vi "Host.vi"() -> ()   [LabVIEW 2013]
uses:
  <vilib>/userdefined/High Color/nirio_resource_hc.ctl
  <instrlib>/niDCPower/nidcpower.llb/niDCPower Measurement Type.ctl
  <vilib>/FPGAPlugInAG/PXI-7953R/niLvFpga_Open_PXI-7953R.vi
  <vilib>/rvi/interface/common/dynamic/niFpgaDynamicAddResources.vi
  <vilib>/FPGAPlugInAG/Dynamic/niLvFpga_Reset_Dynamic.vi
  <vilib>/FPGAPlugInAG/Dynamic/niLvFpga_Run_Dynamic.vi
  <vilib>/rvi/interface/common/niFpgaWaitOnOcc.vi
  <vilib>/Utility/error.llb/Error Cluster From Error Code.vi
  <vilib>/rvi/errors/niLvFpgaAdjustHostInterfaceError.vi
  <vilib>/FPGAPlugInAG/Dynamic/niLvFpga_Close_Dynamic.vi
  <vilib>/rvi/interface/nirviOpenFPGA/nirviOpenFPGA.xnode
  FPGA Bitfiles/MUX1_FPGATarget_Target_25MmX6rN+ac.lvbitx
  <vilib>/rvi/interface/nirviMethod/nirviMethod.xnode
  <vilib>/rvi/interface/nirviReadWriteControl/nirviReadWriteControl.xnode
  <vilib>/rvi/interface/nirviCloseFPGA/nirviCloseFPGA.xnode
  NiFpgaLv.dll
  <vilib>/rvi/interface/Simulation/niFpgaSimulationCallBeginRW.vi
panel:
  in  "100мс до бита":u32=100
  out "СБОЙ":bool
  out "Тиристор":bool
  out "СБОИ":i32
  out "S2":bool
  out "S1":bool
  out "S0":bool
  in  "Контроль S":bool
  in  "VR_ON":bool=TRUE
  out "TST":bool
  out "VDD":i32
  out "VDD3":i32
  out "VDDO":i32
  out "VR":i32
  out "VDDA":i32
  in  "VDD3_selcur":dbl=0.04 caption="current limit" format="%_6p"
  in  "RN":bool
  in  "Автомат":bool
  out "VR":bool
  in  "SEL_Time, мс":u32=100
  in  "SIM_SEL":bool
  in  "VDDA_selcur":dbl=0.04 caption="current limit" format="%_6p"
  in  "VR_selcur":dbl=0.04 caption="current limit" format="%_6p"
  in  "VDDO_selcur":dbl=0.04 caption="current limit" format="%_6p"
  in  "VDD_selcur":dbl=0.04 caption="current limit" format="%_6p"
  in  "VDDA":dbl=3.3 caption="voltage level" format="%_6p"
  in  "VDD3":dbl=3.3 caption="voltage level" format="%_6p"
  in  "VDDA_curlim":dbl=0.05 caption="current limit" format="%_6p"
  in  "VR_curlim":dbl=0.05 caption="current limit" format="%_6p"
  in  "VDD3_curlim":dbl=0.05 caption="current limit" format="%_6p"
  in  "VDD_curlim":dbl=0.05 caption="current limit" format="%_6p"
  out "VDDA_cur":dbl caption="measurement" format="%_6g"
  out "VR_cur":dbl caption="measurement" format="%_6g"
  out "VDD3_cur":dbl caption="measurement" format="%_6g"
  out "VDD_cur":dbl caption="measurement" format="%_6g"
  in  "VR":dbl=3.0 caption="voltage level" format="%_6p"
  in  "VDD":dbl=1.3999999999999997 caption="voltage level" format="%_6p"
  in  "VDDO":dbl=3.3 caption="voltage level" format="%_6p"
  in  "VDDO_curlim":dbl=0.05 caption="current limit" format="%_6p"
  out "VDDO_cur":dbl caption="measurement" format="%_6g"
  out "VDDA":bool
  out "VDDO":bool
  out "VDD3":bool
  out "VDD":bool
  in  "Питание":bool
  in  "Стоп":bool
  in  "VDDA_VR":refnum<k15>="PXI2Slot2" caption="instrument handle"
  in  "VDDO_VDD3":refnum<k15>="PXI1Slot3" caption="instrument handle"
  in  "VDD":refnum<k15>="PXI1Slot4" caption="instrument handle"
  in  "resource name":T1="PXI1Slot5"
  in  "SEL_SEU":path=path "C:/VPL/LabView_PRJ/MUX_1 Folder/VPL/LabView_PRJ/Мультиплексор_2/LOGS"
  out "Номер образца":string="0"
  out "Температура":string="0"
  out "S2":i16
  out "S1":i16
  out "S0":i16
  # "ПЛИС"
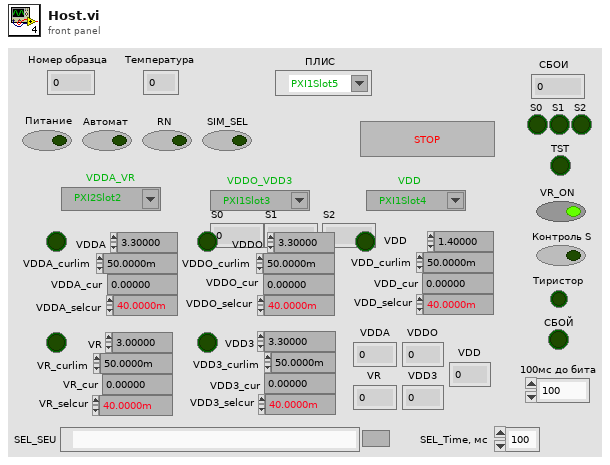
[diagram p1: front panel]
types:
  T1 = typedef "nirio_resource_hc.ctl" = tag
  T2 = enum16{"open", "replace", "create", "open or create", "replace or create", "replace or create with confirmation"}
  T3 = typedef "niDCPower Measurement Type.ctl" = i32
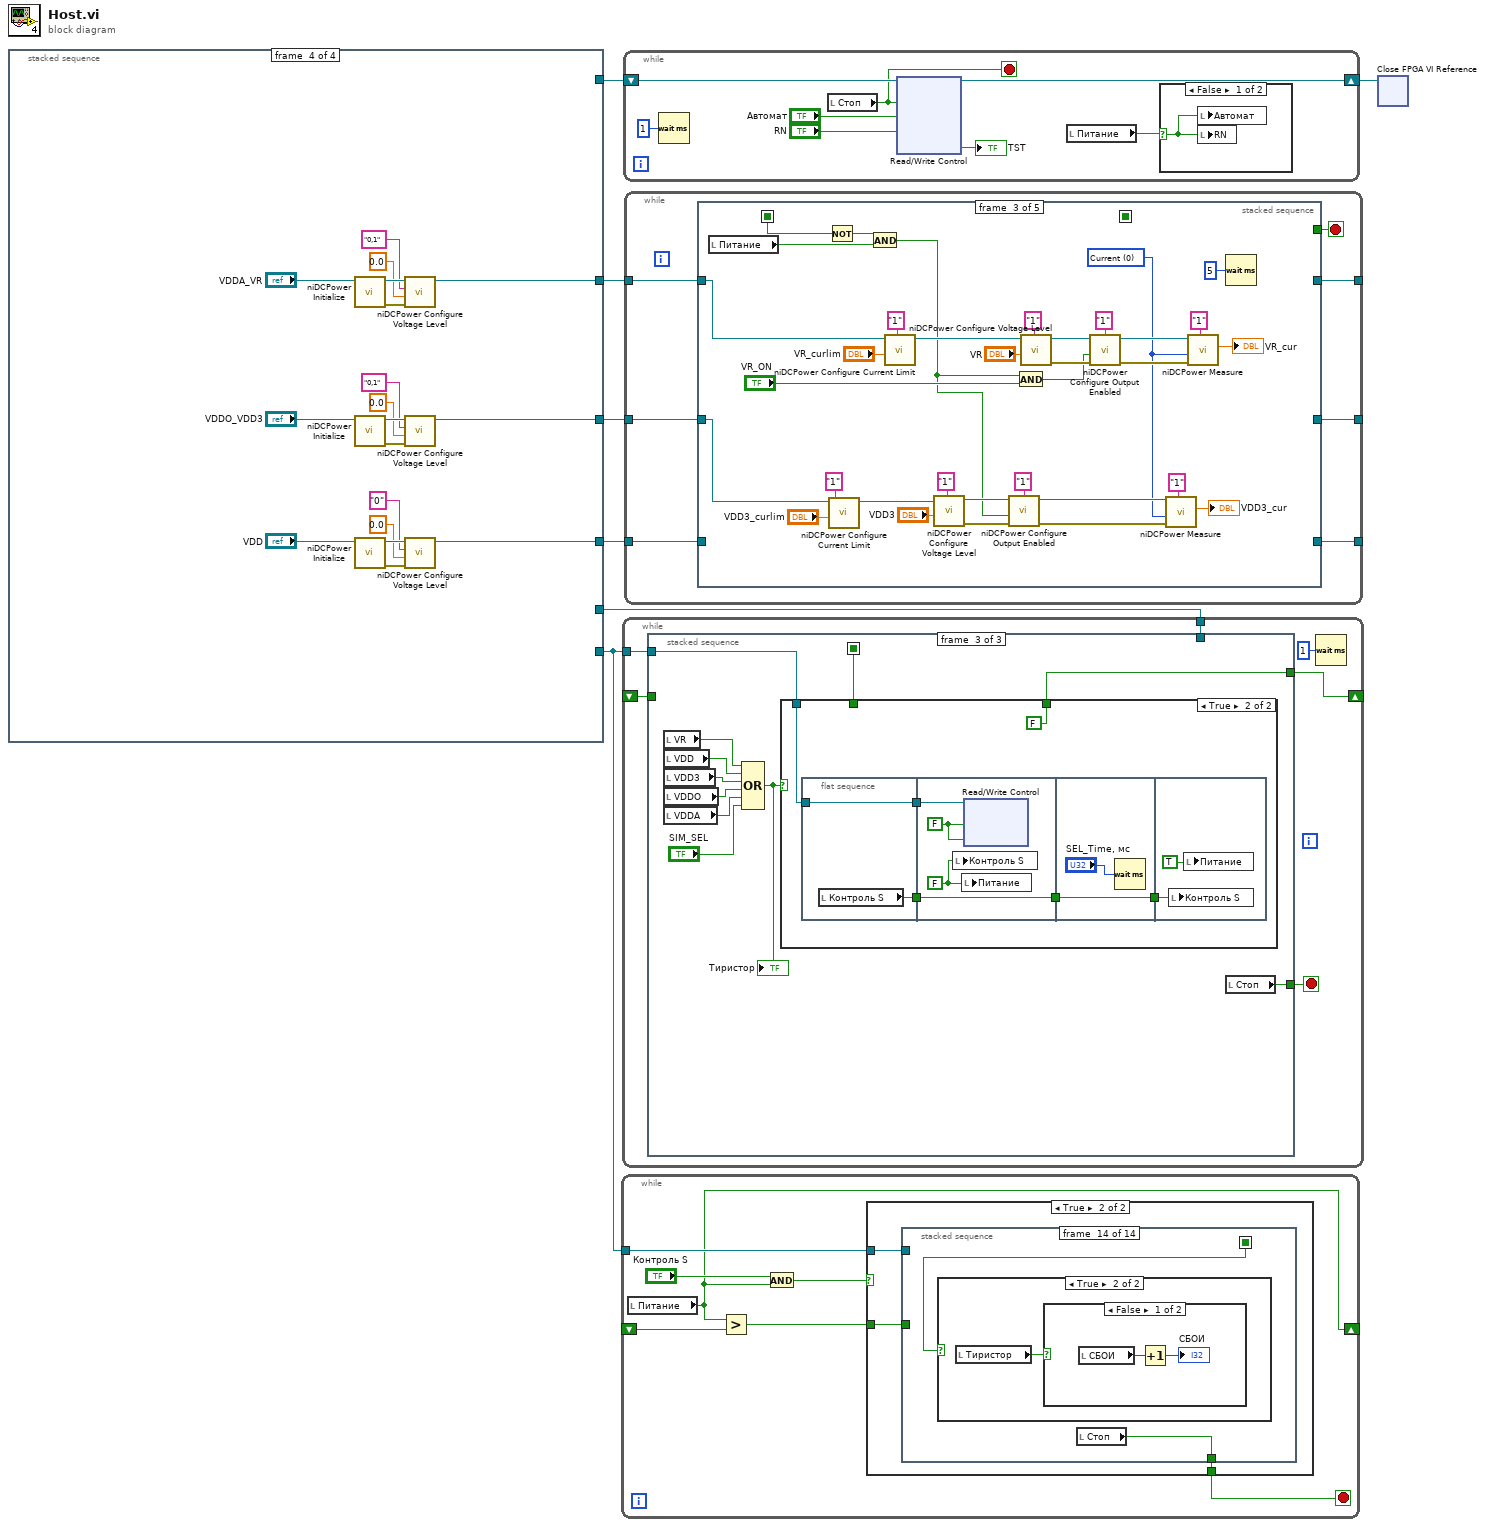
[diagram p0: block diagram]
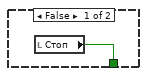
[diagram p2: hidden frame]
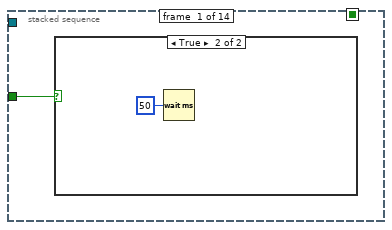
[diagram p3: hidden frame]
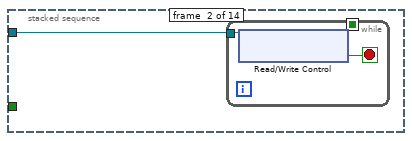
[diagram p5: hidden frame]
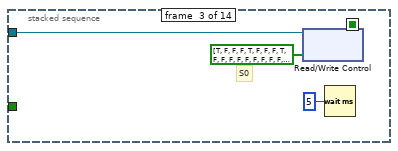
[diagram p6: hidden frame]
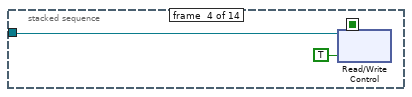
[diagram p7: hidden frame]
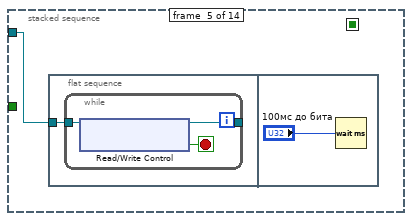
[diagram p8: hidden frame]
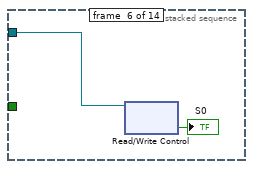
[diagram p9: hidden frame]
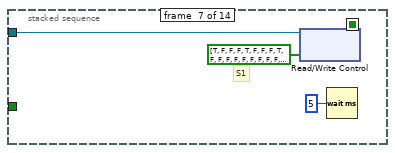
[diagram p10: hidden frame]
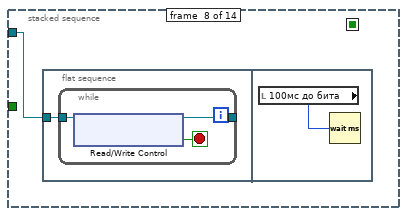
[diagram p11: hidden frame]
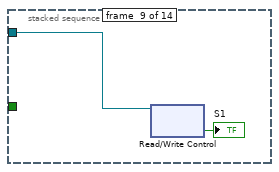
[diagram p12: hidden frame]
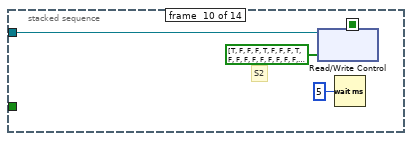
[diagram p13: hidden frame]
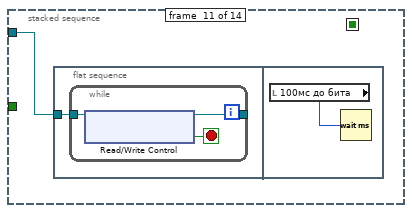
[diagram p14: hidden frame]
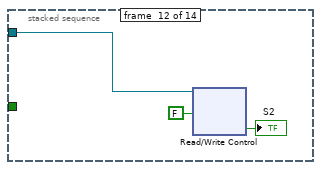
[diagram p15: hidden frame]
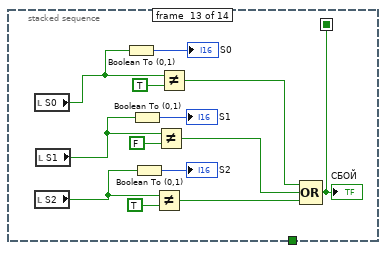
[diagram p16: hidden frame]
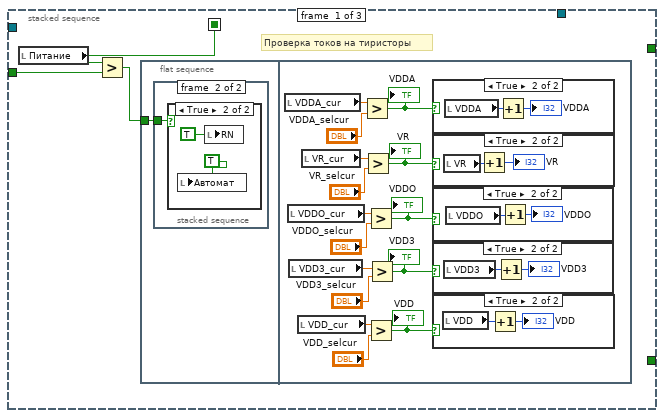
[diagram p20: hidden frame]
diagram:
  n1 = stacked-sequence {
    tunnel: [_ _ w64 _] -> w3
    tunnel: [_ _ _ w72] -> w7
    tunnel: [_ _ _ w71] -> w5
    tunnel: [_ _ _ w70] -> w6
    tunnel: [_ w19 _ _] -> w4
    tunnel: [_ _ w64 _] -> w1
    frame #0 {
      w9 = 0
      w8 = FALSE
      # "Обнуление сбоев"
      # "Обнуление тиристоров"
      # "Отжатие всех кнопок управления"
      n2 = call "Begin.vi"() -> ("Температура 2"=→"Температура":string, "Номер образца 2"=→"Номер образца":string)  [unwired: 10 in]
      n3 = local write "СБОИ"(w9) -> ()
      n4 = local write "VDDA"(w9) -> ()
      n5 = local write "VR"(w9) -> ()
      n6 = local write "VDDO"(w9) -> ()
      n7 = local write "VDD3"(w9) -> ()
      n8 = local write "VDD"(w9) -> ()
      n9 = local write "S1"(w9) -> ()
      n10 = local write "S2"(w9) -> ()
      n11 = local write "S0"(w9) -> ()
      n12 = local write "VR"(w8) -> ()
      n13 = local write "VDD"(w8) -> ()
      n14 = local write "VDD3"(w8) -> ()
      n15 = local write "VDDO"(w8) -> ()
      n16 = local write "VDDA"(w8) -> ()
      n17 = local write "Питание"(w8) -> ()
      n18 = local write "Стоп"(w8) -> ()
      n19 = local write "Автомат"(w8) -> ()
      n20 = local write "RN"(w8) -> ()
      n21 = local write "Контроль S"(w8) -> ()
      n22 = local write "S0"(w8) -> ()
      n23 = local write "S1"(w8) -> ()
      n24 = local write "S2"(w8) -> ()
    }
    frame #1 {
      w14 = "\t"
      n25 = local read "Номер образца"() -> (w48:string)
      n26 = Build Path(base path="SEL_SEU", name or relative path=w48) -> (appended path=w50:path)
      n27 = Get Date/Time In Seconds() -> (seconds since 1Jan1904=w40:timestamp)
      n28 = call <vilib>:"Check if File or Folder Exists.vi"("path"=w50) -> ("file or folder exists?"=w51:bool, "dup path"=w52:path)  [unwired: 8 in, 1 out]
      n29 = Format Date/Time String(time format string (%c)="%d %H.%M.%S", seconds (now)=w40) -> (date/time string=w37:string)  [unwired: 1 in]
      n30 = local read "Температура"() -> (w45:string)
      n31 = case shown="False" w51 {
        tunnel: w52 -> [w61 w62]
        tunnel: [w60 w62] -> w46
        frame False {
          n32 = Create Folder(path (use dialog)=w61) -> (created path=w60:path)  [unwired: 2 in, 2 out]
        }
        frame True {
        }
      }
      n33 = Concatenate Strings(w37, ".xls" ("string")) -> (w35:string)
      n34 = Build Path(base path=w46, name or relative path=w45) -> (appended path=w32:path)
      n35 = call <vilib>:"Check if File or Folder Exists.vi"("path"=w32) -> ("file or folder exists?"=w31:bool, "dup path"=w47:path)  [unwired: 8 in, 1 out]
      n36 = case shown="False" w31 {
        tunnel: w47 -> [w58 w59]
        tunnel: [w57 w59] -> w34
        frame False {
          n37 = Create Folder(path (use dialog)=w58) -> (created path=w57:path)  [unwired: 2 in, 2 out]
        }
        frame True {
        }
      }
      n38 = Build Path(base path=w34, name or relative path=w35) -> (appended path=w38:path)
      n39 = Open/Create/Replace File(file path (use dialog)=w38, operation (0:open)=T2."open or create", access (0:read/write)=enum16{"read/write", "read-only", "write-only"}."read/write") -> (refnum out=w41:refnum<file>)  [unwired: 3 in, 2 out]
      n40 = case shown="True" TRUE {
        tunnel: w41 -> [w53 w56]
        tunnel: [w53 w54] -> w33
        frame False {
        }
        frame True {
          n41 = Set File Position(refnum=w56, from (0:start)=enum16{"start", "end", "current"}."end") -> (refnum out=w54:refnum<file>)  [unwired: 2 in, 1 out]
        }
      }
      n42 = Format Into String(initial string=w33, "Time" ("input 1"), w14, "VDD_cur" ("input 1"), w14, "VDD3_cur" ("input 1"), w14, "VDDO_cur" ("input 1"), w14, "VDDA_cur" ("input 1"), w14, "VR_cur" ("input 1"), w14, "VDD_sel" ("input 1"), w14, "VDD3_sel" ("input 1"), w14, "VDDO_sel" ("input 1"), w14, "VDDA_sel" ("input 1"), w14, "VR_sel" ("input 1"), w14, "Тиристор" ("input 1"), w14, "Всего сбоев" ("input 3"), w14, "S0" ("input 5"), w14, "S1" ("input 7"), w14, "S2" ("input 9"), "\r\n") -> (resulting string=w19:refnum<file>)  [unwired: 2 in, 1 out]
    }
    frame #2 {
      w63 = FALSE
      n43 = xnode "Open FPGA VI Reference"("resource name"="resource name") -> ("FPGA VI Reference Out"=w69:refnum<k20>, "error out"=w67:errorcluster)  [unwired: 1 in]
      n44 = xnode "Invoke Method"("FPGA VI Reference In"=w69, "error in"=w67) -> ("FPGA VI Reference Out"=w66:refnum<k20>, "error out"=w68:errorcluster)
      n45 = xnode "Invoke Method"("FPGA VI Reference In"=w66, "error in"=w68) -> ("FPGA VI Reference Out"=w64:refnum<k20>)  [unwired: 1 in, 1 out]
      n46 = xnode "Read/Write Control"("FPGA VI Reference In"=w64, "Стоп"=w63, "Автомат"=w63, "RN"=w63) -> ()  [unwired: 1 in, 2 out]
    }
    frame #3 {
      n47 = call <instrlib>:"niDCPower Initialize.vi"("resource name"="VDDA_VR") -> ("error out"=w82:errorcluster, "instrument handle out"=w85:refnum<k15>)  [unwired: 3 in, 6 out]
      n48 = call <instrlib>:"niDCPower Initialize.vi"("resource name"="VDDO_VDD3") -> ("error out"=w83:errorcluster, "instrument handle out"=w86:refnum<k15>)  [unwired: 3 in, 6 out]
      n49 = call <instrlib>:"niDCPower Initialize.vi"("resource name"="VDD") -> ("error out"=w84:errorcluster, "instrument handle out"=w87:refnum<k15>)  [unwired: 3 in, 6 out]
      n50 = call <instrlib>:"niDCPower Configure Voltage Level.vi"("error in (no error)"=w82, "voltage level"=0.0, "channel name"="0,1", "instrument handle"=w85) -> ("instrument handle out"=w72:refnum<k15>)  [unwired: 6 in, 1 out]
      n51 = call <instrlib>:"niDCPower Configure Voltage Level.vi"("error in (no error)"=w83, "voltage level"=0.0, "channel name"="0,1", "instrument handle"=w86) -> ("instrument handle out"=w71:refnum<k15>)  [unwired: 6 in, 1 out]
      n52 = call <instrlib>:"niDCPower Configure Voltage Level.vi"("error in (no error)"=w84, "voltage level"=0.0, "channel name"="0", "instrument handle"=w87) -> ("instrument handle out"=w70:refnum<k15>)  [unwired: 6 in, 1 out]
    }
  }
  n53 = while {
    tunnel: w1 -> [w94]
    shift-right: [w90] -> _
    shift-left: _ -> [w91]
    stop <- w88 stop-if-true
    n54 = local read "Питание"() -> (w90:bool)
    n55 = Greater?(x=w90, y=w91) -> (0:w89:bool)
    n56 = And(x="Контроль S", y=w90) -> (x .and. y?=w92:bool)
    n57 = case shown="True" w92 {
      tunnel: w94 -> [_ w98]
      tunnel: w89 -> [_ w97]
      tunnel: [w95 w96] -> w88
      frame False {
        n58 = local read "Стоп"() -> (w95:bool)
      }
      frame True {
        n59 = stacked-sequence {
          seq-local: [_ _ _ _ _ _ _ _ _ _ _ _ w140 _] -> [_ _ _ _ _ _ _ _ _ _ _ _ _ w154]
          tunnel: w98 -> [_ w101 w106 w108 w109 w115 w118 w120 w126 w129 w131 w137 _ _]
          tunnel: w97 -> [w99 _ _ _ _ _ _ _ _ _ _ _ _ _]
          tunnel: [_ _ _ _ _ _ _ _ _ _ _ _ _ w153] -> w96
          frame #0 {
            n60 = case shown="True" w99 {
              frame False {
              }
              frame True {
                n61 = Wait (ms)(milliseconds to wait=u32 50) -> ()  [unwired: 1 out]
              }
            }
          }
          frame #1 {
            n62 = while {
              tunnel: w101 -> [w103]
              stop <- w102 stop-if-true
              n63 = xnode "Read/Write Control"("FPGA VI Reference In"=w103) -> ("Конец посылки?"=w102:bool)  [unwired: 1 in, 2 out]
            }
          }
          frame #2 {
            # "S0"
            n64 = xnode "Read/Write Control"("FPGA VI Reference In"=w106, "SERDAT"=bool[] [TRUE, FALSE, FALSE, FALSE, TRUE, FALSE, FALSE, FALSE, TRUE, FALSE, FALSE, FALSE, FALSE, FALSE, FALSE, FALSE, FALSE, FALSE, FALSE, FALSE, FALSE, TRUE, TRUE, TRUE, TRUE, TRUE, TRUE, TRUE, TRUE, FALSE]) -> ()  [unwired: 1 in, 2 out]
            n65 = Wait (ms)(milliseconds to wait=u32 5) -> ()  [unwired: 1 out]
          }
          frame #3 {
            n66 = xnode "Read/Write Control"("FPGA VI Reference In"=w108, "S_start"=TRUE) -> ()  [unwired: 1 in, 2 out]
          }
          frame #4 {
            n67 = flat-sequence {
              tunnel: w109 -> [w110]
              frame #0 {
                n68 = while {
                  tunnel: w110 -> [w113]
                  tunnel: [w111] -> _
                  stop <- w112 stop-if-true
                  n69 = xnode "Read/Write Control"("FPGA VI Reference In"=w113) -> ("FPGA VI Reference Out"=w111:refnum<k20>, "Конец посылки?"=w112:bool)  [unwired: 1 in, 1 out]
                }
              }
              frame #1 {
                n70 = Wait (ms)(milliseconds to wait="100мс до бита") -> ()  [unwired: 1 out]
              }
            }
          }
          frame #5 {
            n71 = xnode "Read/Write Control"("FPGA VI Reference In"=w115) -> ("TST"=→"S0":bool)  [unwired: 1 in, 2 out]
          }
          frame #6 {
            # "S1"
            n72 = xnode "Read/Write Control"("FPGA VI Reference In"=w118, "SERDAT"=bool[] [TRUE, FALSE, FALSE, FALSE, TRUE, FALSE, FALSE, FALSE, TRUE, FALSE, FALSE, FALSE, FALSE, FALSE, FALSE, FALSE, FALSE, FALSE, FALSE, TRUE, FALSE, TRUE, TRUE, TRUE, TRUE, TRUE, TRUE, TRUE, TRUE, FALSE]) -> ()  [unwired: 1 in, 2 out]
            n73 = Wait (ms)(milliseconds to wait=u32 5) -> ()  [unwired: 1 out]
          }
          frame #7 {
            n74 = flat-sequence {
              tunnel: w120 -> [w121]
              frame #0 {
                n75 = while {
                  tunnel: w121 -> [w124]
                  tunnel: [w122] -> _
                  stop <- w123 stop-if-true
                  n76 = xnode "Read/Write Control"("FPGA VI Reference In"=w124) -> ("FPGA VI Reference Out"=w122:refnum<k20>, "Конец посылки?"=w123:bool)  [unwired: 1 in, 1 out]
                }
              }
              frame #1 {
                n77 = local read "100мс до бита"() -> (w125:u32)
                n78 = Wait (ms)(milliseconds to wait=w125) -> ()  [unwired: 1 out]
              }
            }
          }
          frame #8 {
            n79 = xnode "Read/Write Control"("FPGA VI Reference In"=w126) -> ("TST"=→"S1":bool)  [unwired: 1 in, 2 out]
          }
          frame #9 {
            # "S2"
            n80 = xnode "Read/Write Control"("FPGA VI Reference In"=w129, "SERDAT"=bool[] [TRUE, FALSE, FALSE, FALSE, TRUE, FALSE, FALSE, FALSE, TRUE, FALSE, FALSE, FALSE, FALSE, FALSE, FALSE, FALSE, FALSE, FALSE, TRUE, FALSE, FALSE, TRUE, TRUE, TRUE, TRUE, TRUE, TRUE, TRUE, TRUE, FALSE]) -> ()  [unwired: 1 in, 2 out]
            n81 = Wait (ms)(milliseconds to wait=u32 5) -> ()  [unwired: 1 out]
          }
          frame #10 {
            n82 = flat-sequence {
              tunnel: w131 -> [w132]
              frame #0 {
                n83 = while {
                  tunnel: w132 -> [w135]
                  tunnel: [w133] -> _
                  stop <- w134 stop-if-true
                  n84 = xnode "Read/Write Control"("FPGA VI Reference In"=w135) -> ("FPGA VI Reference Out"=w133:refnum<k20>, "Конец посылки?"=w134:bool)  [unwired: 1 in, 1 out]
                }
              }
              frame #1 {
                n85 = local read "100мс до бита"() -> (w136:u32)
                n86 = Wait (ms)(milliseconds to wait=w136) -> ()  [unwired: 1 out]
              }
            }
          }
          frame #11 {
            n87 = xnode "Read/Write Control"("FPGA VI Reference In"=w137, "S_start"=FALSE) -> ("TST"=→"S2":bool)  [unwired: 1 in, 2 out]
          }
          frame #12 {
            n88 = local read "S0"() -> (w149:bool)
            n89 = local read "S2"() -> (w143:bool)
            n90 = local read "S1"() -> (w146:bool)
            n91 = Boolean To (0,1)(Boolean=w149) -> (0, 1=→"S0":i16)
            n92 = Boolean To (0,1)(Boolean=w146) -> (0, 1=→"S1":i16)
            n93 = Boolean To (0,1)(Boolean=w143) -> (0, 1=→"S2":i16)
            n94 = Not Equal?(x=w143, y=TRUE) -> (x != y?=w141:bool)
            n95 = Not Equal?(x=w146, y=FALSE) -> (x != y?=w144:bool)
            n96 = Not Equal?(x=w149, y=TRUE) -> (x != y?=w147:bool)
            n97 = Compound Arithmetic op=OR(w147, w144, w141) -> (w140:bool)
            "СБОЙ" <- w140
          }
          frame #13 {
            n98 = case shown="True" w154 {
              frame False {
              }
              frame True {
                n99 = local read "Тиристор"() -> (w155:bool)
                n100 = case shown="False" w155 {
                  frame False {
                    n101 = local read "СБОИ"() -> (w157:i32)
                    n102 = Increment(x=w157) -> (x+1=→"СБОИ":i32)
                  }
                  frame True {
                  }
                }
              }
            }
            n103 = local read "Стоп"() -> (w153:bool)
          }
        }
      }
    }
  }
  n104 = while {
    tunnel: w4 -> [w162]
    shift-right: [w158] -> _
    shift-left: _ -> [w161]
    tunnel: w1 -> [w160]
    stop <- w159 stop-if-true
    n105 = stacked-sequence {
      seq-local: [w164 _ _] -> [_ _ w250]
      tunnel: w162 -> [_ w246 _]
      tunnel: [_ _ w249] -> w158
      tunnel: w161 -> [w166 _ _]
      tunnel: w160 -> [_ _ w258]
      tunnel: [_ _ w251] -> w159
      frame #0 {
        # "Проверка токов на тиристоры"
        n106 = local read "Питание"() -> (w164:bool)
        n107 = Greater?(x=w164, y=w166) -> (0:w165:bool)
        n108 = flat-sequence {
          tunnel: w165 -> [w167]
          frame #0 {
            n109 = stacked-sequence {
              tunnel: w167 -> [w168 w170]
              frame #0 {
                n110 = case shown="True" w168 {
                  frame False {
                  }
                  frame True {
                    n111 = Wait (ms)(milliseconds to wait=u32 100) -> ()  [unwired: 1 out]
                  }
                }
              }
              frame #1 {
                n112 = case shown="True" w170 {
                  frame False {
                  }
                  frame True {
                    n113 = local write "Автомат"(TRUE ("RN")) -> ()
                    n114 = local write "RN"(TRUE ("RN")) -> ()
                  }
                }
              }
            }
          }
          frame #1 {
            n115 = local read "VDDA_cur"() -> (w182:dbl)
            n116 = local read "VDDO_cur"() -> (w180:dbl)
            n117 = local read "VDD3_cur"() -> (w179:dbl)
            n118 = local read "VDD_cur"() -> (w178:dbl)
            n119 = local read "VR_cur"() -> (w181:dbl)
            n120 = Greater?(x=w182, y="VDDA_selcur") -> (0:w175:bool)
            "VDDA" <- w175
            n121 = Greater?(x=w181, y="VR_selcur") -> (0:w176:bool)
            "VR" <- w176
            n122 = Greater?(x=w180, y="VDDO_selcur") -> (0:w173:bool)
            "VDDO" <- w173
            n123 = Greater?(x=w178, y="VDD_selcur") -> (0:w177:bool)
            "VDD" <- w177
            n124 = Greater?(x=w179, y="VDD3_selcur") -> (0:w174:bool)
            "VDD3" <- w174
            n125 = case shown="True" w175 {
              frame False {
              }
              frame True {
                n126 = local read "VDDA"() -> (w197:i32)
                n127 = Increment(x=w197) -> (x+1=→"VDDA":i32)
              }
            }
            n128 = case shown="True" w176 {
              frame False {
              }
              frame True {
                n129 = local read "VR"() -> (w195:i32)
                n130 = Increment(x=w195) -> (x+1=→"VR":i32)
              }
            }
            n131 = case shown="True" w173 {
              frame False {
              }
              frame True {
                n132 = local read "VDDO"() -> (w193:i32)
                n133 = Increment(x=w193) -> (x+1=→"VDDO":i32)
              }
            }
            n134 = case shown="True" w174 {
              frame False {
              }
              frame True {
                n135 = local read "VDD3"() -> (w191:i32)
                n136 = Increment(x=w191) -> (x+1=→"VDD3":i32)
              }
            }
            n137 = case shown="True" w177 {
              frame False {
              }
              frame True {
                n138 = local read "VDD"() -> (w189:i32)
                n139 = Increment(x=w189) -> (x+1=→"VDD":i32)
              }
            }
          }
        }
      }
      frame #1 {
        w208 = i16 0 ("width (-)")
        w209 = i16 0 ("width (-)")
        w210 = i16 0 ("width (-)")
        w211 = i16 0 ("width (-)")
        w233 = i16 0 ("width (-)")
        w234 = i16 3 ("width (-)")
        w203 = "\t"
        n140 = local read "VDDO_cur"() -> (w230:dbl)
        n141 = local read "VDDA_cur"() -> (w229:dbl)
        n142 = local read "VDD3_cur"() -> (w231:dbl)
        n143 = local read "VDD_cur"() -> (w232:dbl)
        n144 = local read "SIM_SEL"() -> (w242:bool)
        n145 = local read "VR_cur"() -> (w228:dbl)
        n146 = local read "VDDO"() -> (w225:i32)
        n147 = local read "VDDA"() -> (w224:i32)
        n148 = local read "VDD3"() -> (w226:i32)
        n149 = local read "VDDO"() -> (w235:bool)
        n150 = local read "VDDA"() -> (w237:bool)
        n151 = local read "VDD3"() -> (w236:bool)
        n152 = local read "VDD"() -> (w227:i32)
        n153 = local read "VDD"() -> (w238:bool)
        n154 = local read "VR"() -> (w223:i32)
        n155 = local read "VR"() -> (w239:bool)
        n156 = Number To Fractional String(number=w232, width (-)=w234, precision (6)=w234) -> (F-format string=w222:string)  [unwired: 1 in]
        n157 = Number To Fractional String(number=w231, width (-)=w234, precision (6)=w234) -> (F-format string=w221:string)  [unwired: 1 in]
        n158 = Number To Fractional String(number=w230, width (-)=w234, precision (6)=w234) -> (F-format string=w220:string)  [unwired: 1 in]
        n159 = Number To Fractional String(number=w229, width (-)=w234, precision (6)=w234) -> (F-format string=w219:string)  [unwired: 1 in]
        n160 = Number To Fractional String(number=w228, width (-)=w234, precision (6)=w234) -> (F-format string=w218:string)  [unwired: 1 in]
        n161 = Number To Fractional String(number=w227, width (-)=w233, precision (6)=w233) -> (F-format string=w217:string)  [unwired: 1 in]
        n162 = Number To Fractional String(number=w226, width (-)=w233, precision (6)=w233) -> (F-format string=w216:string)  [unwired: 1 in]
        n163 = Number To Fractional String(number=w225, width (-)=w233, precision (6)=w233) -> (F-format string=w215:string)  [unwired: 1 in]
        n164 = Number To Fractional String(number=w224, width (-)=w233, precision (6)=w233) -> (F-format string=w214:string)  [unwired: 1 in]
        n165 = Number To Fractional String(number=w223, width (-)=w233, precision (6)=w233) -> (F-format string=w213:string)  [unwired: 1 in]
        n166 = Compound Arithmetic op=OR(w239, w238, w237, w236, w235, w242) -> (w240:bool)
        n167 = Get Date/Time In Seconds() -> (seconds since 1Jan1904=w248:timestamp)
        n168 = Select(t="!!!", s=w240, f="") -> (s? t:f=w212:string)
        n169 = Format Date/Time String(time format string (%c)="%d %H:%M:%S:%3u", seconds (now)=w248) -> (date/time string=w241:string)  [unwired: 1 in]
        n170 = local read "СБОИ"() -> (w207:i32)
        n171 = local read "S0"() -> (w206:i16)
        n172 = local read "S2"() -> (w204:i16)
        n173 = local read "S1"() -> (w205:i16)
        n174 = Number To Fractional String(number=w207, width (-)=w211, precision (6)=w211) -> (F-format string=w201:string)  [unwired: 1 in]
        n175 = Number To Fractional String(number=w206, width (-)=w210, precision (6)=w210) -> (F-format string=w200:string)  [unwired: 1 in]
        n176 = Number To Fractional String(number=w205, width (-)=w209, precision (6)=w209) -> (F-format string=w199:string)  [unwired: 1 in]
        n177 = Number To Fractional String(number=w204, width (-)=w208, precision (6)=w208) -> (F-format string=w198:string)  [unwired: 1 in]
        n178 = Concatenate Strings(w241, w203, w222, w203, w221, w203, w220, w203, w219, w203, w218, w203, w217, w203, w216, w203, w215, w203, w214, w203, w213, w203, w212, w203, w201, w203, w200, w203, w199, w203, w198, "\r\n") -> (w247:string)
        n179 = Format Into String(initial string=w246, w247) -> ()  [unwired: 2 in, 2 out]
      }
      frame #2 {
        n180 = local read "VR"() -> (w252:bool)
        n181 = local read "VDD"() -> (w253:bool)
        n182 = local read "VDD3"() -> (w254:bool)
        n183 = local read "VDDO"() -> (w255:bool)
        n184 = local read "VDDA"() -> (w256:bool)
        n185 = Compound Arithmetic op=OR(w252, w253, w254, w255, w256, "SIM_SEL") -> (w257:bool)
        "Тиристор" <- w257
        n186 = case shown="True" w257 {
          tunnel: w258 -> [_ w266]
          tunnel: w250 -> [w260 _]
          tunnel: [w260 FALSE] -> w249
          frame False {
          }
          frame True {
            n187 = flat-sequence {
              tunnel: w266 -> [w268]
              tunnel: [w268] -> w264
              tunnel: [w267] -> w261
              tunnel: w264 -> [w272]
              tunnel: [w269] -> w262
              tunnel: w261 -> [w269]
              tunnel: [w273] -> w263
              tunnel: w262 -> [w273]
              tunnel: w263 -> [w275]
              frame #0 {
                n188 = local read "Контроль S"() -> (w267:bool)
              }
              frame #1 {
                w270 = FALSE ("SYS_RESET")
                w271 = FALSE ("SYS_RESET")
                n189 = local write "Контроль S"(w270) -> ()
                n190 = local write "Питание"(w270) -> ()
                n191 = xnode "Read/Write Control"("FPGA VI Reference In"=w272, "Автомат"=w271, "RN"=w271) -> ()  [unwired: 1 in, 2 out]
              }
              frame #2 {
                n192 = Wait (ms)(milliseconds to wait="SEL_Time, мс") -> ()  [unwired: 1 out]
              }
              frame #3 {
                n193 = local write "Контроль S"(w275) -> ()
                n194 = local write "Питание"(TRUE ("SYS_RESET")) -> ()
              }
            }
          }
        }
        n195 = local read "Стоп"() -> (w251:bool)
      }
    }
    n196 = Wait (ms)(milliseconds to wait=u32 1) -> ()  [unwired: 1 out]
  }
  n197 = while {
    shift-right: [w283] -> w2
    shift-left: w3 -> [w284]
    stop <- w278 stop-if-true
    n198 = Wait (ms)(milliseconds to wait=u32 1) -> ()  [unwired: 1 out]
    n199 = local read "Стоп"() -> (w278:bool)
    n200 = xnode "Read/Write Control"("FPGA VI Reference In"=w284, "Стоп"=w278, "Автомат"="Автомат", "RN"="RN") -> ("FPGA VI Reference Out"=w283:refnum<k20>, "TST"=→"TST":bool)  [unwired: 1 in, 1 out]
    n201 = local read "Питание"() -> (w280:bool)
    n202 = case shown="False" w280 {
      selector: w280 -> [w285 _]
      frame False {
        n203 = local write "Автомат"(w285) -> ()
        n204 = local write "RN"(w285) -> ()
      }
      frame True {
      }
    }
  }
  n205 = while {
    tunnel: w6 -> [w292]
    tunnel: w5 -> [w291]
    tunnel: w7 -> [w290]
    tunnel: [w288] -> _
    tunnel: [w287] -> _
    tunnel: [w286] -> _
    stop <- w289 stop-if-true
    n206 = stacked-sequence {
      seq-local: ["Стоп" _ _ _ _] -> [_ w298 w331 w364 _]
      seq-local: ["Стоп" _ _ _ _] -> [_ w297 _ _ _]
      tunnel: w292 -> [_ _ _ w366 w380]
      tunnel: w291 -> [_ w302 w328 _ w381]
      tunnel: w290 -> [_ w301 w333 _ w382]
      tunnel: [_ w297 _ _ _] -> w289
      tunnel: [_ _ _ _ w382] -> w288
      tunnel: [_ _ _ _ w381] -> w287
      tunnel: [_ _ _ _ w380] -> w286
      frame #0 {
      }
      frame #1 {
        w294 = T3 0 items=["Current", "Voltage"] ("measurement type")
        n207 = Wait (ms)(milliseconds to wait=u32 5) -> ()  [unwired: 1 out]
        n208 = Not(x=w298) -> (.not. x?=w300:bool)
        n209 = And(x=w300, y="Питание") -> (x .and. y?=w296:bool)
        n210 = call <instrlib>:"niDCPower Configure Current Limit.vi"("current limit"="VDDA_curlim", "channel name"="0", "instrument handle"=w301) -> ("instrument handle out"=w321:refnum<k15>)  [unwired: 7 in, 1 out]
        n211 = call <instrlib>:"niDCPower Configure Current Limit.vi"("current limit"="VDDO_curlim", "channel name"="0", "instrument handle"=w302) -> ("instrument handle out"=w308:refnum<k15>)  [unwired: 7 in, 1 out]
        n212 = call <instrlib>:"niDCPower Configure Voltage Level.vi"("voltage level"="VDDA", "channel name"="0", "instrument handle"=w321) -> ("error out"=w317:errorcluster, "instrument handle out"=w318:refnum<k15>)  [unwired: 7 in]
        n213 = call <instrlib>:"niDCPower Configure Voltage Level.vi"("voltage level"="VDDO", "channel name"="0", "instrument handle"=w308) -> ("error out"=w312:errorcluster, "instrument handle out"=w313:refnum<k15>)  [unwired: 7 in]
        n214 = call <instrlib>:"niDCPower Configure Output Enabled.vi"("error in (no error)"=w317, "output enabled"=w296, "channel name"="0", "instrument handle"=w318) -> ("error out"=w324:errorcluster, "instrument handle out"=w323:refnum<k15>)  [unwired: 6 in]
        n215 = call <instrlib>:"niDCPower Configure Output Enabled.vi"("error in (no error)"=w312, "output enabled"=w296, "channel name"="0", "instrument handle"=w313) -> ("error out"=w304:errorcluster, "instrument handle out"=w305:refnum<k15>)  [unwired: 6 in]
        n216 = call <instrlib>:"niDCPower Measure.vi"("error in (no error)"=w324, "measurement type"=w294, "channel name"="0", "instrument handle"=w323) -> ("measurement"=→"VDDA_cur":dbl)  [unwired: 5 in, 2 out]
        n217 = call <instrlib>:"niDCPower Measure.vi"("error in (no error)"=w304, "measurement type"=w294, "channel name"="0", "instrument handle"=w305) -> ("measurement"=→"VDDO_cur":dbl)  [unwired: 5 in, 2 out]
      }
      frame #2 {
        w327 = T3 0 items=["Current", "Voltage"] ("measurement type")
        n218 = local read "Питание"() -> (w330:bool)
        n219 = Not(x=w331) -> (.not. x?=w332:bool)
        n220 = call <instrlib>:"niDCPower Configure Current Limit.vi"("current limit"="VDD3_curlim", "channel name"="1", "instrument handle"=w328) -> ("instrument handle out"=w356:refnum<k15>)  [unwired: 7 in, 1 out]
        n221 = And(x=w332, y=w330) -> (x .and. y?=w329:bool)
        n222 = call <instrlib>:"niDCPower Configure Current Limit.vi"("current limit"="VR_curlim", "channel name"="1", "instrument handle"=w333) -> ("instrument handle out"=w342:refnum<k15>)  [unwired: 7 in, 1 out]
        n223 = call <instrlib>:"niDCPower Configure Voltage Level.vi"("voltage level"="VDD3", "channel name"="1", "instrument handle"=w356) -> ("error out"=w354:errorcluster, "instrument handle out"=w353:refnum<k15>)  [unwired: 7 in]
        n224 = call <instrlib>:"niDCPower Configure Output Enabled.vi"("error in (no error)"=w354, "output enabled"=w329, "channel name"="1", "instrument handle"=w353) -> ("error out"=w359:errorcluster, "instrument handle out"=w358:refnum<k15>)  [unwired: 6 in]
        n225 = And(x=w329, y="VR_ON") -> (x .and. y?=w339:bool)
        n226 = call <instrlib>:"niDCPower Configure Voltage Level.vi"("voltage level"="VR", "channel name"="1", "instrument handle"=w342) -> ("error out"=w340:errorcluster, "instrument handle out"=w341:refnum<k15>)  [unwired: 7 in]
        n227 = call <instrlib>:"niDCPower Configure Output Enabled.vi"("error in (no error)"=w340, "output enabled"=w339, "channel name"="1", "instrument handle"=w341) -> ("error out"=w344:errorcluster, "instrument handle out"=w345:refnum<k15>)  [unwired: 6 in]
        n228 = call <instrlib>:"niDCPower Measure.vi"("error in (no error)"=w359, "measurement type"=w327, "channel name"="1", "instrument handle"=w358) -> ("measurement"=→"VDD3_cur":dbl)  [unwired: 5 in, 2 out]
        n229 = call <instrlib>:"niDCPower Measure.vi"("error in (no error)"=w344, "measurement type"=w327, "channel name"="1", "instrument handle"=w345) -> ("measurement"=→"VR_cur":dbl)  [unwired: 5 in, 2 out]
        n230 = Wait (ms)(milliseconds to wait=u32 5) -> ()  [unwired: 1 out]
      }
      frame #3 {
        w361 = T3 0 items=["Current", "Voltage"] ("measurement type")
        n231 = local read "Питание"() -> (w363:bool)
        n232 = Not(x=w364) -> (.not. x?=w365:bool)
        n233 = call <instrlib>:"niDCPower Configure Current Limit.vi"("current limit"="VDD_curlim", "channel name"="0", "instrument handle"=w366) -> ("instrument handle out"=w374:refnum<k15>)  [unwired: 7 in, 1 out]
        n234 = And(x=w365, y=w363) -> (x .and. y?=w362:bool)
        n235 = Wait (ms)(milliseconds to wait=u32 5) -> ()  [unwired: 1 out]
        n236 = call <instrlib>:"niDCPower Configure Voltage Level.vi"("voltage level"="VDD", "channel name"="0", "instrument handle"=w374) -> ("error out"=w372:errorcluster, "instrument handle out"=w373:refnum<k15>)  [unwired: 7 in]
        n237 = call <instrlib>:"niDCPower Configure Output Enabled.vi"("error in (no error)"=w372, "output enabled"=w362, "channel name"="0", "instrument handle"=w373) -> ("error out"=w377:errorcluster, "instrument handle out"=w376:refnum<k15>)  [unwired: 6 in]
        n238 = call <instrlib>:"niDCPower Measure.vi"("error in (no error)"=w377, "measurement type"=w361, "channel name"="0", "instrument handle"=w376) -> ("measurement"=→"VDD_cur":dbl)  [unwired: 5 in, 2 out]
      }
      frame #4 {
      }
    }
  }
  n239 = xnode "Close FPGA VI Reference"("FPGA VI Reference In"=w2) -> ()  [unwired: 1 in, 1 out]
